vi "Session4_StateMachine.vi"() -> ()   [LabVIEW 2016]
panel:
  in  "milliseconds to wait":u32=200
  out "Thermometer":dbl(slide) scale=0.0..100.0
  out "Temp Value":dbl
  in  "Clear":bool
  out "Temp Chart":dbl(graph)
  in  "Sensor Simulator":dbl(slide) scale=0.0..100.0
  in  "stop":bool
  # "Session 4 – Project: State Machine for Real-Time Temperature Display"
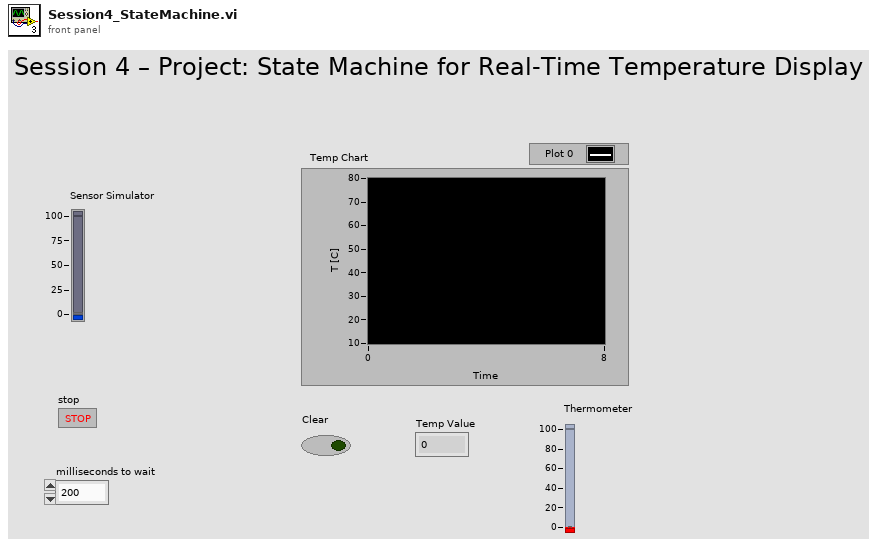
[diagram p1: front panel]
types:
  T1 = enum16{"Initialize", "IDLE", "Clear Chart", "Update Chart"}
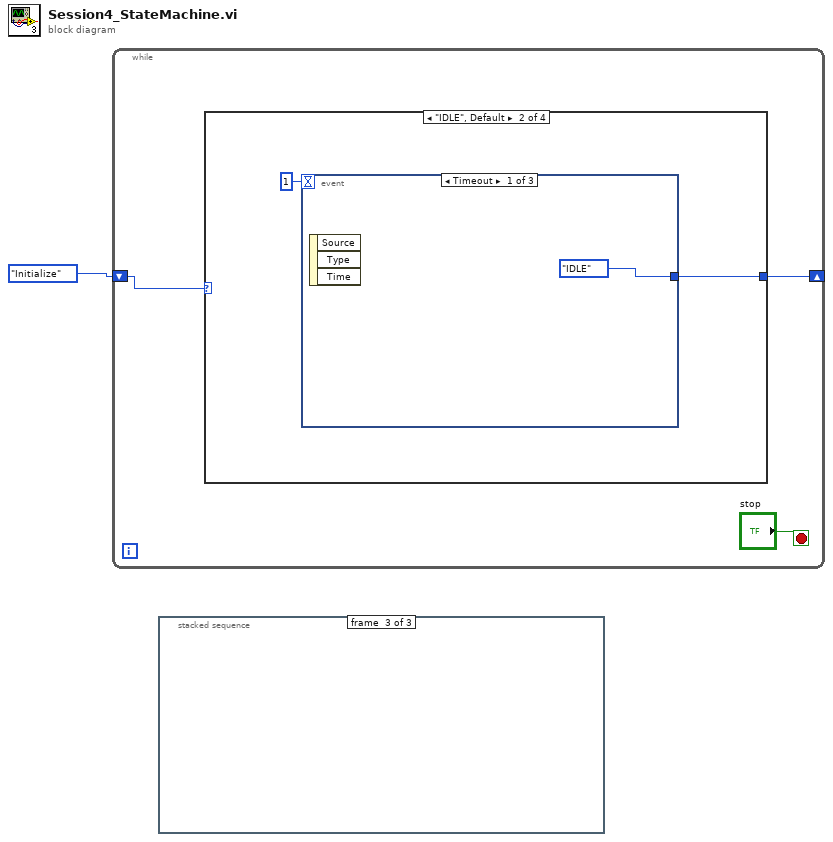
[diagram p0: block diagram]
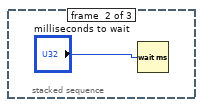
[diagram p3: hidden frame]
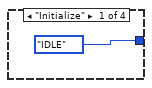
[diagram p4: hidden frame]
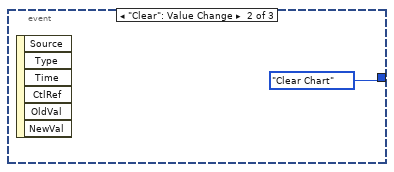
[diagram p5: hidden frame]
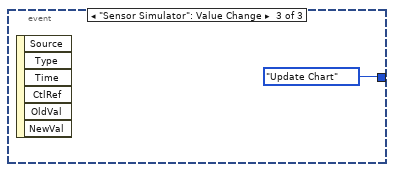
[diagram p6: hidden frame]
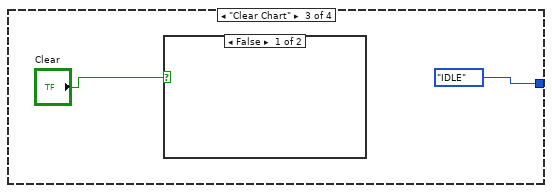
[diagram p7: hidden frame]
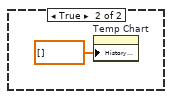
[diagram p8: hidden frame]
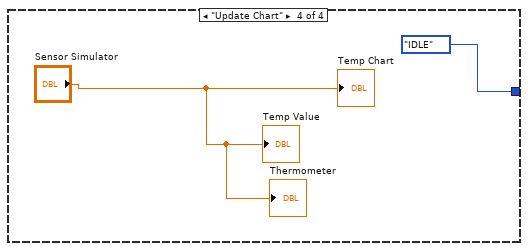
[diagram p9: hidden frame]
diagram:
  n1 = while {
    shift-right: [w2] -> _
    shift-left: T1."Initialize" -> [w3]
    stop <- "stop" stop-if-true
    n2 = case shown="\"IDLE\", Default" w3 {
      tunnel: [T1."IDLE" w6 T1."IDLE" T1."IDLE"] -> w2
      frame "Initialize" {
      }
      frame "IDLE", Default {
        n3 = event shown="[0] Timeout" {
          selector: _ -> [_ _ _]
          dyn-events: _ -> [_ _ _]
          timeout: 1 -> [_ _ _]
          tunnel: [T1."IDLE" T1."Clear Chart" T1."Update Chart"] -> w6
          event Timeout {
            n4 = event-data() -> ()  [unwired: 1 in, 3 out]
          }
          event "Clear": Value Change {
            n5 = event-data() -> ()  [unwired: 1 in, 6 out]
          }
          event "Sensor Simulator": Value Change {
            n6 = event-data() -> ()  [unwired: 1 in, 6 out]
          }
        }
      }
      frame "Clear Chart" {
        n7 = case shown="False" "Clear" {
          frame False {
          }
          frame True {
            n8 = property on="Temp Chart" class="WFChart (strict)"("History Data"=dbl[] []) -> ()  [unwired: 2 in, 2 out]
          }
        }
      }
      frame "Update Chart" {
        "Temp Chart" <- "Sensor Simulator"
        "Temp Value" <- "Sensor Simulator"
        "Thermometer" <- "Sensor Simulator"
      }
    }
  }
  n9 = stacked-sequence {
    frame #0 {
    }
    frame #1 {
      n10 = Wait (ms)(milliseconds to wait="milliseconds to wait") -> ()  [unwired: 1 out]
    }
    frame #2 {
    }
  }
